vi "Write Card Arr Ref.vi"(8 "error in (no error)":errorcluster, 10 "Card Arr Ref":refnum<vi>, 11 "Universal Power Meter in":refnum<class "Universal Power Meter.lvclass">) -> (0 "error out":errorcluster, 3 "Universal Power Meter out":refnum<class "Universal Power Meter.lvclass">)   [LabVIEW 2012, in "Universal Power Meter.lvlib" / "Universal Power Meter.lvclass"]
uses:
  Universal Power Meter.lvclass
  Universal Power Meter.lvclass/Universal Power Meter.ctl
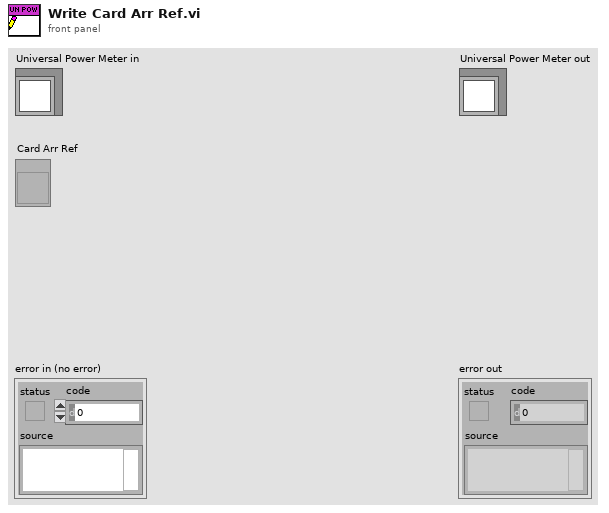
[diagram p1: front panel]
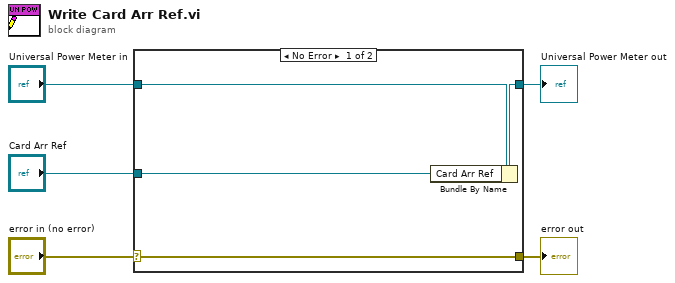
[diagram p0: block diagram]
diagram:
  n1 = case shown="No Error" "error in (no error)" {
    selector: "error in (no error)" -> [w9 w10]
    tunnel: [w9 w10] -> w4
    tunnel: [w7 w11] -> w2
    tunnel: "Universal Power Meter in" -> [w8 w11]
    tunnel: "Card Arr Ref" -> [w6 _]
    frame No Error {
      n2 = Bundle By Name(cluster=w8, "Card Arr Ref"=w6) -> (w7:refnum<class "Universal Power Meter.lvclass">)
    }
    frame Error {
    }
  }
  "error out" <- w4
  "Universal Power Meter out" <- w2
